vi "ActionVIOnRecompile.vi"(8 "error in":errorcluster, 10 "node_path":string, 11 "Device Item Ref in":T1 format="%.0x") -> (0 "error out":errorcluster)   [LabVIEW 2025, in "Runtime Configuration Support Example System Explorer.lvlib"]
uses:
  Runtime Configuration Support Example System Explorer.lvlib
  <vilib>/NI VeriStand/Custom Device API/Custom Device Item Ref.ctl
  <vilib>/NI VeriStand/Custom Device API/Custom Device Channel Type.ctl
  Shared/Compiled.Settings.ctl
  <vilib>/NI VeriStand/Custom Device API/Data Access Type.ctl
  <vilib>/NI VeriStand/Custom Device API/Get Item Property (I32).vi
  Error Constants.vi
  <vilib>/NI VeriStand/Execution/CustomDevice/NI VeriStand - Send Custom Device Message (Byte Array).vi
  <vilib>/NI VeriStand/Custom Device API/Custom Device API.lvlib
  Shared/Runtime Configuration Support Example Shared.lvlib
  <vilib>/NI VeriStand/execution/CustomDevice/NI_VS Custom Device ExecutionAPI.lvlib
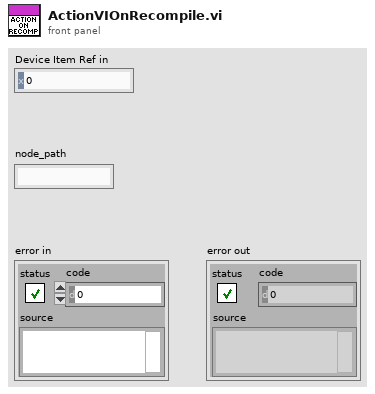
[diagram p1: front panel]
types:
  T1 = typedef "Custom Device API.lvlib/Custom Device Item Ref.ctl" = u64
  T2 = cluster{"Dynamic Config Status":bool, "Inports":i32[], "Outports":i32[], "Error":errorcluster}
  T3 = typedef "Runtime Configuration Support Example Shared.lvlib/Compiled.Settings.ctl" = cluster{"Name":string, "Inport SignalIDs":i32[], "Outport SignalIDs":i32[], "Inport Channel refs":T1[], "Outport Channel refs":T1[], "Inport Values":dbl[], "Outport Values":dbl[], "Device Error":errorcluster, "Dynamic Config Status":bool, "Response Ref":refnum<queue>}
  T4 = typedef "Custom Device API.lvlib/Custom Device Channel Type.ctl" = enum16{"Input", "Output"}
  T5 = typedef "Custom Device API.lvlib/Data Access Type.ctl" = enum16{"Read", "Write"}
  T6 = typedef "Custom Device API.lvlib/Data Reference.ctl" = i32
  T7 = typedef "NI_VS Custom Device ExecutionAPI.lvlib/Custom Device Ref.ctl" = refnum<k24>
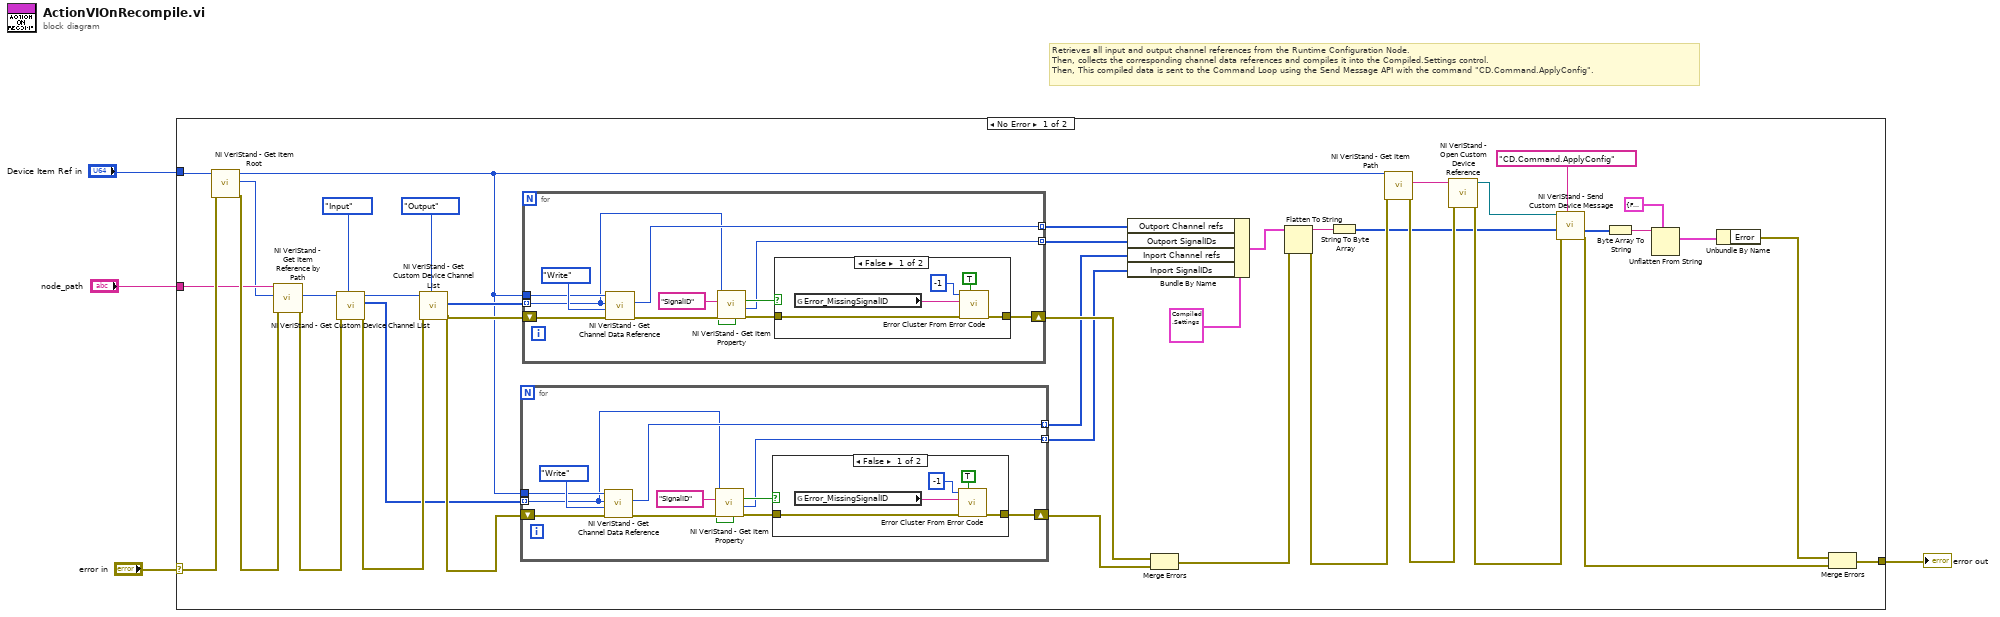
[diagram p0: block diagram]
diagram:
  # "Retrieves all input and output channel references from the Runtime Configuration Node.\nThen, collects the corresponding channel data references and compiles it into the Compiled.Settings control.\nThen, This compiled data is sent to the Command Loop using the Send Message API with the command \"CD.Command.ApplyConfig\"."
  n1 = case shown="No Error" "error in" {
    selector: "error in" -> [w36 w78]
    tunnel: [w30 w78] -> w3
    tunnel: "Device Item Ref in" -> [w24 _]
    tunnel: "node_path" -> [w25 _]
    frame No Error {
      n2 = call <vilib>:"NI VeriStand - Get Item Root.vi"("error in (no error)"=w36, "Item Ref in"=w24) -> ("error out"=w40:errorcluster, "Root Ref out"=w23:T1, "Item Ref out"=w12:T1)  [unwired: 6 in, 1 out]
      n3 = call <vilib>:"NI VeriStand - Get Item Reference by Path.vi"("error in (no error)"=w40, "Root Ref"=w23, "Item Path in"=w25) -> ("error out"=w39:errorcluster, "Item Ref"=w21:T1)  [unwired: 5 in, 2 out]
      n4 = call <vilib>:"NI VeriStand - Get Custom Device Channel List.vi"("Channel Type"=Custom_Device_Channel_Type."Input", "error in (no error)"=w39, "Device Ref in"=w21) -> ("error out"=w43:errorcluster, "Specified Channel Ref List"=w11:T1[], "Device Ref out"=w22:T1)  [unwired: 6 in]
      n5 = call <vilib>:"NI VeriStand - Get Custom Device Channel List.vi"("Channel Type"=Custom_Device_Channel_Type."Output", "error in (no error)"=w43, "Device Ref in"=w22) -> ("error out"=w35:errorcluster, "Specified Channel Ref List"=w19:T1[])  [unwired: 6 in, 1 out]
      n6 = for {
        tunnel: w11 -> [w47] mode=indexing
        shift-right: [w51] -> w34
        shift-left: w35 -> [w54]
        tunnel: w12 -> [w49]
        tunnel: [w48] -> w10 mode=indexing
        tunnel: [w44] -> w9 mode=indexing
        n7 = call <vilib>:"NI VeriStand - Get Channel Data Reference.vi"("error in (no error)"=w54, "Access"=Data_Access_Type."Write", "Channel Ref in"=w47, "Device Ref in"=w49) -> ("error out"=w53:errorcluster, "Channel Data Reference"=w48:T6)  [unwired: 5 in, 1 out]
        n8 = call-poly <vilib>:"NI VeriStand - Get Item Property.vi"("error in (no error)"=w53, "Property Name"="SignalID", "Item Ref in"=w47) -> ("error out"=w52:errorcluster, "Value"=w44:i32, "Found?"=w45:bool)  [unwired: 5 in, 1 out]
        n9 = case shown="False" w45 {
          tunnel: w52 -> [w59 w60]
          tunnel: [w58 w60] -> w51
          frame False {
            n10 = global read "Error Constants.vi" "Error_MissingSignalID"() -> (w55:string)
            n11 = call <vilib>:"Error Cluster From Error Code.vi"("show call chain? (False)"=TRUE, "error in (no error)"=w59, "error message (\"\")"=w55, "error code (0)"=-1) -> ("error out"=w58:errorcluster)  [unwired: 5 in]
          }
          frame True {
          }
        }
      }
      n12 = for {
        tunnel: w19 -> [w64] mode=indexing
        shift-right: [w68] -> w37
        shift-left: w35 -> [w71]
        tunnel: w12 -> [w66]
        tunnel: [w65] -> w15 mode=indexing
        tunnel: [w61] -> w14 mode=indexing
        n13 = call <vilib>:"NI VeriStand - Get Channel Data Reference.vi"("error in (no error)"=w71, "Access"=Data_Access_Type."Write", "Channel Ref in"=w64, "Device Ref in"=w66) -> ("error out"=w70:errorcluster, "Channel Data Reference"=w65:T6)  [unwired: 5 in, 1 out]
        n14 = call-poly <vilib>:"NI VeriStand - Get Item Property.vi"("error in (no error)"=w70, "Property Name"="SignalID", "Item Ref in"=w64) -> ("error out"=w69:errorcluster, "Value"=w61:i32, "Found?"=w62:bool)  [unwired: 5 in, 1 out]
        n15 = case shown="False" w62 {
          tunnel: w69 -> [w76 w77]
          tunnel: [w75 w77] -> w68
          frame False {
            n16 = global read "Error Constants.vi" "Error_MissingSignalID"() -> (w72:string)
            n17 = call <vilib>:"Error Cluster From Error Code.vi"("show call chain? (False)"=TRUE, "error in (no error)"=w76, "error message (\"\")"=w72, "error code (0)"=-1) -> ("error out"=w75:errorcluster)  [unwired: 5 in]
          }
          frame True {
          }
        }
      }
      n18 = Bundle By Name(cluster=T3 {"Name"="", "Inport SignalIDs"=[], "Outport SignalIDs"=[], "Inport Channel refs"=[], "Outport Channel refs"=[], "Inport Values"=[], "Outport Values"=[], "Device Error"={"status"=FALSE, "code"=0, "source"=""}, "Dynamic Config Status"=FALSE, "Response Ref"=refnum} ("Compiled.Settings"), "Outport Channel refs"=w15, "Outport SignalIDs"=w14, "Inport Channel refs"=w10, "Inport SignalIDs"=w9) -> (w13:T3)
      n19 = Merge Errors(w37, w34) -> (w33:errorcluster)
      n20 = Flatten To String(anything=w13, error in (no error)=w33) -> (data string=w17:string, error out=w42:errorcluster)  [unwired: 2 in, 1 out]
      n21 = String To Byte Array(string=w17) -> (unsigned byte array=w16:u8[])
      n22 = call <vilib>:"NI VeriStand - Get Item Path.vi"("error in (no error)"=w42, "Item Ref in"=w12) -> ("error out"=w41:errorcluster, "Path"=w26:string)  [unwired: 6 in, 2 out]
      n23 = call <vilib>:"NI VeriStand - Open Custom Device Reference.vi"("error in (no error)"=w41, "Custom Device Path"=w26) -> ("error out"=w38:errorcluster, "Custom Device"=w20:T7)  [unwired: 8 in]
      n24 = call-poly <vilib>:"NI VeriStand - Send Custom Device Message.vi"("error in (no error)"=w38, "Data"=w16, "Command"="CD.Command.ApplyConfig", "Custom Device in"=w20) -> ("error out"=w32:errorcluster, "Response"=w8:u8[])  [unwired: 5 in, 1 out]
      n25 = Byte Array To String(unsigned byte array=w8) -> (string=w7:string)
      n26 = Unflatten From String(type=T2 {"Dynamic Config Status"=FALSE, "Inports"=[], "Outports"=[], "Error"={"status"=FALSE, "code"=0, "source"=""}}, binary string=w7) -> (value=w6:T2)  [unwired: 3 in, 2 out]
      n27 = Unbundle By Name(w6) -> ("Error"=w31:errorcluster)
      n28 = Merge Errors(w31, w32) -> (w30:errorcluster)
    }
    frame Error {
    }
  }
  "error out" <- w3
